vi "cavity_model_wrapper.vi"(0 "Data in":fxp<+/-,32,14>[](array[numeric])=[0.0, 0.0, 0.0, 0.0], 2 "enabled":bool=TRUE, 3 "virtual cavity":bool=TRUE, 5 "input valid":bool=TRUE, 6 "reset":bool=TRUE, 7 "C3":fxp<+/-,32,3>=-2.180195599794388 format="%#_30g", 8 "C1":fxp<+/-,32,1>=0.9986428320407867, 9 "C4":fxp<+/-,32,1>=0.999985234811902, 10 "C2":fxp<+/-,32,3>=0.002117181196808815 format="%#_30g", 11 "C5":fxp<+/-,32,-32>=-5.4752209710517974e-18 format="%#_60g") -> (14 "Data out":fxp<+/-,32,14>[](array[numeric]), 16 "Ai1 out":fxp<+/-,32,14>[](array[numeric]), 19 "output valid":bool)   [LabVIEW 2018]
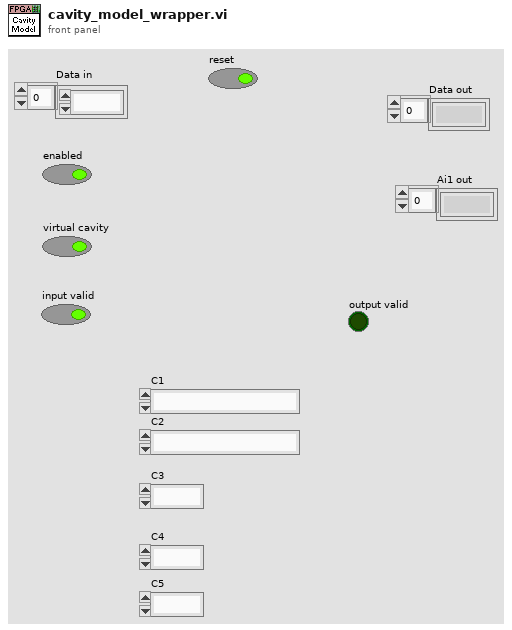
[diagram p1: front panel]
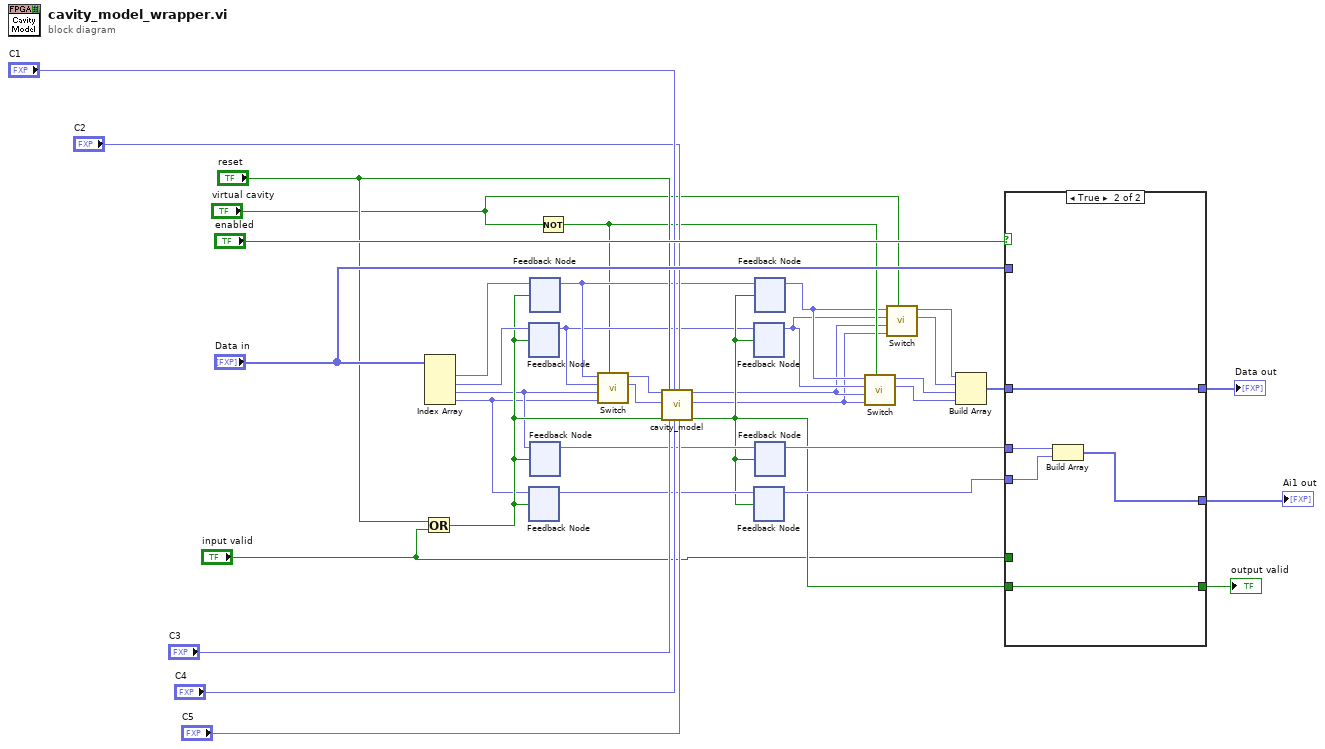
[diagram p0: block diagram]
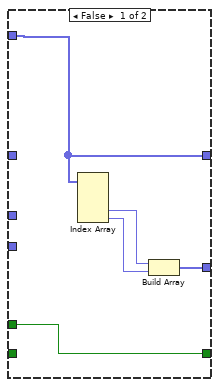
[diagram p2: hidden frame]
diagram:
  n1 = Or(x="reset", y="input valid") -> (x .or. y?=w17:bool)
  n2 = Index Array(array="Data in") -> (element #1=w26:fxp<+/-,32,14>, element #2=w25:fxp<+/-,32,14>, element #3=w16:fxp<+/-,32,14>, element #4=w15:fxp<+/-,32,14>)  [unwired: 4 in]
  n3 = feedback #1() -> (w13:fxp<+/-,32,14>)  [unwired: 1 in]
  n4 = feedback-in #1(w25, w17) -> ()
  n5 = feedback #2() -> (w22:fxp<+/-,32,14>)  [unwired: 1 in]
  n6 = feedback-in #2(w15, w17) -> ()
  n7 = feedback #3() -> (w14:fxp<+/-,32,14>)  [unwired: 1 in]
  n8 = feedback-in #3(w26, w17) -> ()
  n9 = feedback #4() -> (w24:fxp<+/-,32,14>)  [unwired: 1 in]
  n10 = feedback-in #4(w16, w17) -> ()
  n11 = Not(x="virtual cavity") -> (.not. x?=w8:bool)
  n12 = call "Switch.vi"("Use Ch0"=w8, "Ch1 Q"=w15, "Ch1 I"=w16, "Ch0 Q"=w13, "Ch0 I"=w14) -> ("Out Q"=w12:fxp<+/-,32,14>, "Out I"=w11:fxp<+/-,32,14>)  [unwired: 5 in]
  n13 = call "cavity_model.vi"("Ir"=w11, "Ii"=w12, "input valid"=w17, "reset"="reset", "C3"="C3", "C1"="C1", "C4"="C4", "C2"="C2", "C5"="C5") -> ("Vr"=w2:fxp<+/-,32,14>, "Vi"=w1:fxp<+/-,32,14>, "output valid"=w20:bool)  [unwired: 8 in]
  n14 = feedback #5() -> (w6:fxp<+/-,32,14>)  [unwired: 1 in]
  n15 = feedback-in #5(w13, w20) -> ()
  n16 = feedback #6() -> (w21:fxp<+/-,32,14>)  [unwired: 1 in]
  n17 = feedback-in #6(w22, w20) -> ()
  n18 = feedback #7() -> (w7:fxp<+/-,32,14>)  [unwired: 1 in]
  n19 = feedback-in #7(w14, w20) -> ()
  n20 = feedback #8() -> (w23:fxp<+/-,32,14>)  [unwired: 1 in]
  n21 = feedback-in #8(w24, w20) -> ()
  n22 = call "Switch.vi"("Use Ch0"=w8, "Ch1 Q"=w1, "Ch1 I"=w2, "Ch0 Q"=w6, "Ch0 I"=w7) -> ("Out Q"=w9:fxp<+/-,32,14>, "Out I"=w10:fxp<+/-,32,14>)  [unwired: 5 in]
  n23 = call "Switch.vi"("Use Ch0"="virtual cavity", "Ch1 Q"=w1, "Ch1 I"=w2, "Ch0 Q"=w6, "Ch0 I"=w7) -> ("Out Q"=w4:fxp<+/-,32,14>, "Out I"=w5:fxp<+/-,32,14>)  [unwired: 5 in]
  n24 = Build Array(w5, w4, w10, w9) -> (w37:fxp<+/-,32,14>[])
  n25 = case shown="True" "enabled" {
    tunnel: w37 -> [_ w47]
    tunnel: [w40 w47] -> w36
    tunnel: w20 -> [_ w46]
    tunnel: [w42 w46] -> w34
    tunnel: "Data in" -> [w40 _]
    tunnel: "input valid" -> [w42 _]
    tunnel: [w41 w43] -> w32
    tunnel: w23 -> [_ w45]
    tunnel: w21 -> [_ w44]
    frame False {
      n26 = Index Array(array=w40) -> (element #3=w39:fxp<+/-,32,14>, element #4=w38:fxp<+/-,32,14>)  [unwired: 4 in, 2 out]
      n27 = Build Array(w39, w38) -> (w41:fxp<+/-,32,14>[])
    }
    frame True {
      n28 = Build Array(w45, w44) -> (w43:fxp<+/-,32,14>[])
    }
  }
  "output valid" <- w34
  "Data out" <- w36
  "Ai1 out" <- w32
